vi "Stop Core.vi"(10 "final error code":i32, 11 "LTI ULS Actor in":refnum<class "LTI ULS Actor.lvclass">) -> (3 "LTI ULS Actor out":refnum<class "LTI ULS Actor.lvclass">)   [LabVIEW 2018, in "LTI ULS Actor.lvlib" / "LTI ULS Actor.lvclass"]
doc: "In addition to the following, this method also sends a message to the monitor to notify it that the actor has stopped execution.\n\n(<B>Filename</B>: Actor Framework.lvlib:Actor.lvclass:Stop Core.vi)\n\nDefines what the actor does before it stops. Use the <B>final error code</B> input to determine whether the actor shut down in response to an error.\n\nBy default, this method does nothing. A descendant class may override it to define behavior, such as shutting down any processes the actor initiated in its override of the Actor Core method.\n\nCopyright: MGI\nAuthored by: Derek Trepanier"
uses:
  LTI ULS Actor.lvclass
  C:/Users/dev/Documents/CODE/LabVIEW/microwaveverify/trunk/MWWL Verification/Sensor Actor/Sensor/Sensor.lvclass
  LTI ULS Actor.lvclass/LTI ULS Actor.ctl
  Sensor Actor/Sensor/Sensor.lvclass
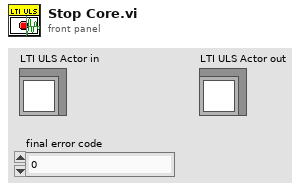
[diagram p1: front panel]
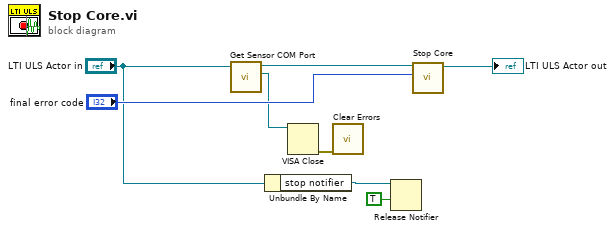
[diagram p0: block diagram]
diagram:
  n1 = call "Get Sensor COM Port.vi"("Sensor in"="LTI ULS Actor in") -> ("COM Port"=w2:refnum<visa-resource-name>, "Sensor out"=w3:refnum<class "LTI ULS Actor.lvclass">)  [unwired: 8 in, 1 out]
  n2 = Unbundle By Name("LTI ULS Actor in") -> ("stop notifier"=w6:refnum<notifier>)
  n3 = VISA Close(VISA resource name=w2) -> (error out=w1:errorcluster)  [unwired: 1 in]
  n4 = call <vilib>:"Clear Errors.vi"("error in (no error)"=w1) -> ()  [unwired: 5 in, 2 out]
  n5 = Release Notifier(notifier=w6, force destroy? (F)=TRUE) -> ()  [unwired: 1 in, 3 out]
  n6 = call-parent "Stop Core.vi"("final error code"="final error code", "Sensor in"=w3) -> ("Sensor out"=→"LTI ULS Actor out":refnum<class "LTI ULS Actor.lvclass">)  [unwired: 9 in]
